vi "Add Employees to Employee Table.vi"(8 "错误输入（无错误）":errorcluster, 10 "Array":T1[](array[typedef]), 11 "DataTable":refnum<k24>) -> (0 "错误输出（无错误）":errorcluster, 3 "DataTable Out":refnum<k24>)   [LabVIEW 2012, in "Employee Info.lvlib"]
uses:
  Employee Info.lvlib
  System.Data
  Employee Info.ctl
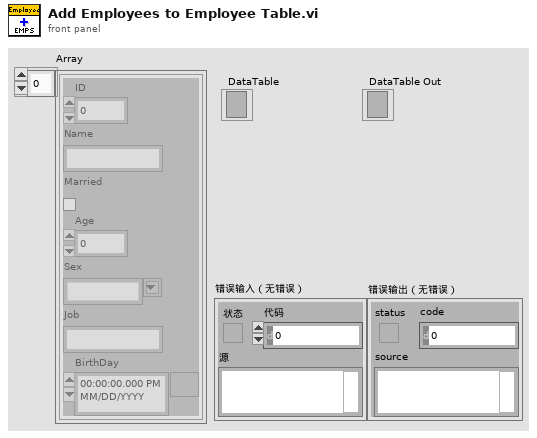
[diagram p1: front panel]
types:
  T1 = typedef "Employee Info.lvlib/Employee Info.ctl" = cluster{"ID":u16, "Name":string, "Married":bool, "Age":u8, "Sex":string, "Job":string, "BirthDay":timestamp}
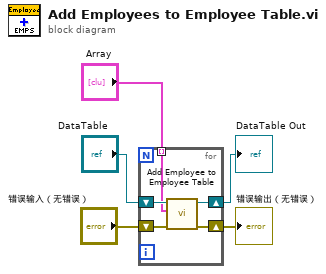
[diagram p0: block diagram]
diagram:
  n1 = for {
    shift-right: [w7] -> w2
    shift-left: "错误输入（无错误）" -> [w8]
    shift-right: [w9] -> w3
    shift-left: "DataTable" -> [w10]
    tunnel: "Array" -> [w6] mode=indexing
    n2 = call "Add Employee to Employee Table.vi"("错误输入（无错误）"=w8, "Employee Info"=w6, "DataTable"=w10) -> ("错误输出"=w7:errorcluster, "DataTable Out"=w9:refnum<k24>)  [unwired: 7 in]
  }
  "DataTable Out" <- w3
  "错误输出（无错误）" <- w2
